vi "multilineStringToArray_3.vi"(3 "multilineString":string) -> (0 "stringArrayDimension":i32, 1 "stringArray":string[](array[string]))   [LabVIEW 2014]
doc: "WARNING: fast routine reserved for UNI_MAG (the character \\b is used as dummy delimiter for the \"Spreadsheet String To Array\" operator).\n\nConverts a dataset multiline string into a string array.\nValid line terminators are \\r and \\n."
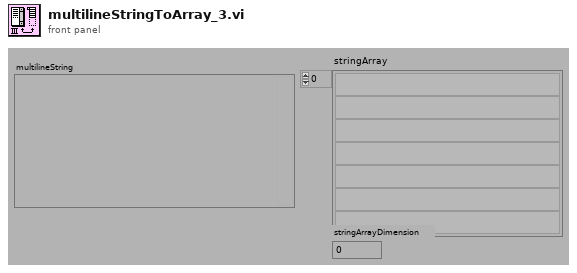
[diagram p1: front panel]
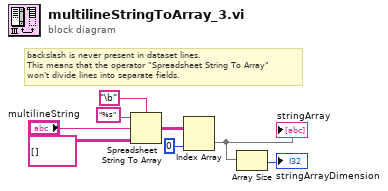
[diagram p0: block diagram]
diagram:
  # "backslash is never present in dataset lines.\nThis means that the operator \"Spreadsheet String To Array\"\nwon't divide lines into separate fields."
  n1 = Spreadsheet String To Array(delimiter (Tab)="\b", format string="%s", spreadsheet string="multilineString", array type (2D Dbl)=string[][] []) -> (array=w1:string[][])
  n2 = Index Array(array=w1, index (col)=0) -> (element=w4:string[])  [unwired: 1 in]
  "stringArray" <- w4
  n3 = Array Size(array=w4) -> (size(s)=→"stringArrayDimension":i32)
